vi "printfilecopy.vi"(11 "源路径":path) -> (2 "copy status":bool, 3 "new path":path)   [LabVIEW 2011]
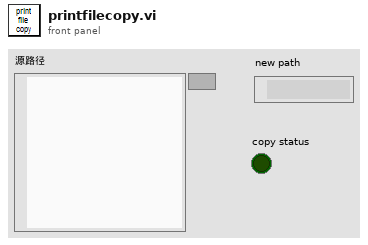
[diagram p1: front panel]
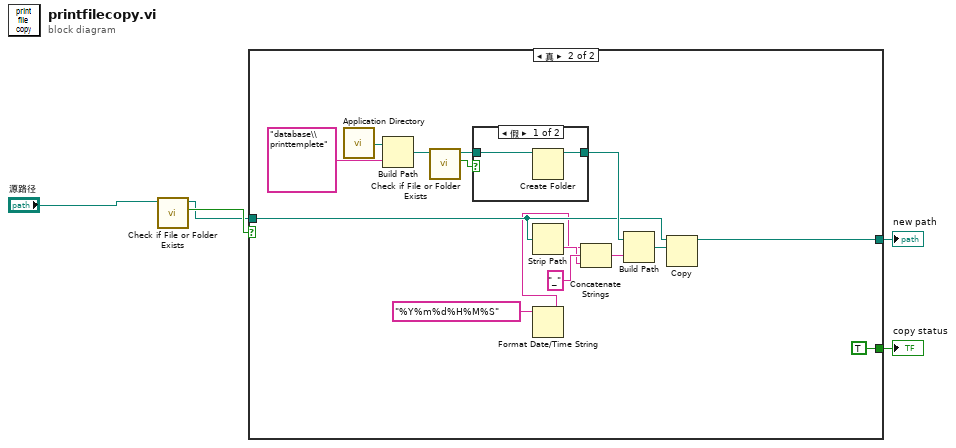
[diagram p0: block diagram]
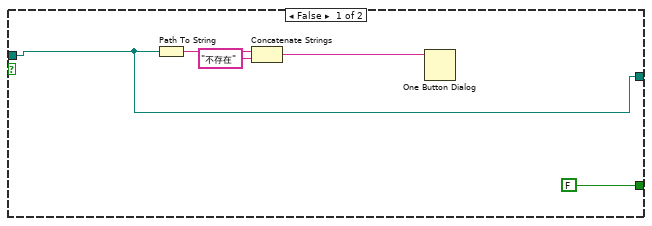
[diagram p2: hidden frame]
diagram:
  n1 = call <vilib>:"Check if File or Folder Exists.vi"("path"="源路径") -> ("file or folder exists?"=w4:bool, "dup path"=w3:path)  [unwired: 8 in, 1 out]
  n2 = case shown="真" w4 {
    tunnel: w3 -> [w7 w15]
    tunnel: [w7 w14] -> w1
    tunnel: [FALSE TRUE] -> w2
    frame False {
      n3 = Path To String(path=w7) -> (string=w10:string)
      n4 = Concatenate Strings(w10, "不存在" ("字符串")) -> (w8:string)
      n5 = One Button Dialog(message=w8) -> ()  [unwired: 1 in, 1 out]
    }
    frame True {
      n6 = call <vilib>:"Application Directory.vi"() -> ("Application Directory"=w25:path)
      n7 = Build Path(base path=w25, name or relative path="database\\printtemplete" ("名称或相对路径")) -> (appended path=w23:path)
      n8 = call <vilib>:"Check if File or Folder Exists.vi"("path"=w23) -> ("file or folder exists?"=w22:bool, "dup path"=w21:path)  [unwired: 8 in, 1 out]
      n9 = case shown="假" w22 {
        tunnel: w21 -> [w27 w28]
        tunnel: [w26 w28] -> w20
        frame False {
          n10 = Create Folder(path (use dialog)=w27) -> (created path=w26:path)  [unwired: 2 in, 2 out]
        }
        frame True {
        }
      }
      n11 = Strip Path(path=w15) -> (name=w12:string)  [unwired: 1 out]
      n12 = Format Date/Time String(time format string (%c)="%Y%m%d%H%M%S" ("时间格式字符串(%c)")) -> (date/time string=w11:string)  [unwired: 2 in]
      n13 = Concatenate Strings(w11, "_" ("字符串"), w12) -> (w17:string)
      n14 = Build Path(base path=w20, name or relative path=w17) -> (appended path=w16:path)
      n15 = Copy(10:w16, 11:w15) -> (3:w14:path)  [unwired: 3 in, 2 out]
    }
  }
  "copy status" <- w2
  "new path" <- w1
